vi "foldersfiles.vi"(4 "error in":errorcluster, 7 "path":path) -> (0 "error out":errorcluster, 1 "Array 2":path[](array[path]), 2 "Array":T1(array[cluster]), 3 "path out":path)   [LabVIEW 2010]
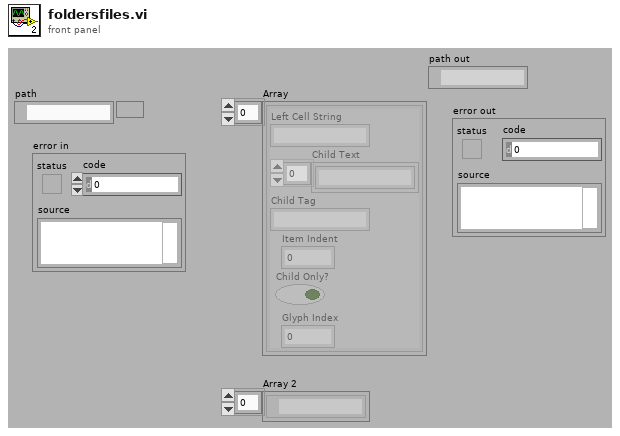
[diagram p1: front panel]
types:
  T1 = cluster{"Left Cell String":string, "Child Text":string[], "Child Tag":string, "Item Indent":i32, "Child Only?":bool, "Glyph Index":i32}[]
  T2 = cluster{"Left Cell String":string, "Child Text":string[], "Child Tag":string, "Item Indent":i32, "Child Only?":bool, "Glyph Index":i32}
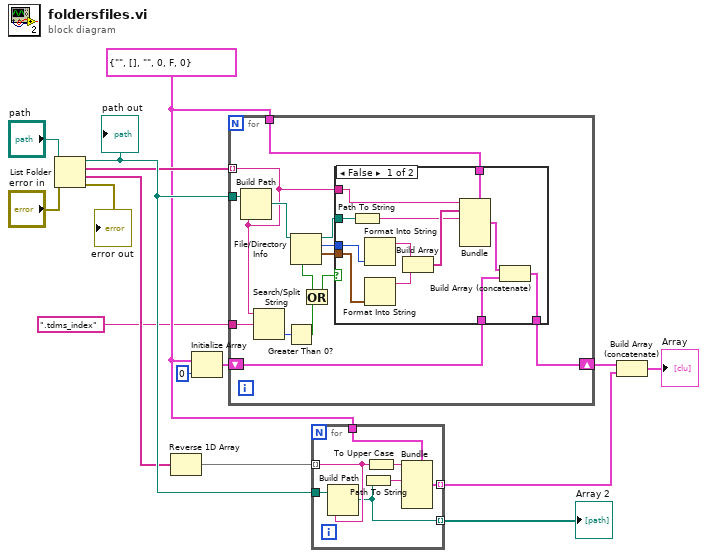
[diagram p0: block diagram]
diagram:
  w4 = T2 {"Left Cell String"="", "Child Text"=[], "Child Tag"="", "Item Indent"=0, "Child Only?"=FALSE, "Glyph Index"=0} ("Item")
  n1 = List Folder(path="path", error in="error in") -> (path out=w14:path, filenames=w6:string[], folder names=w10:string[], error out=→"error out":errorcluster)  [unwired: 2 in]
  "path out" <- w14
  n2 = Reverse 1D Array(array=w10) -> (reversed array=w7:string[])
  n3 = Initialize Array(w4, 0 ("dimension size")) -> (w5:T1)
  n4 = for {
    tunnel: w4 -> [w26]
    tunnel: w6 -> [w23] mode=indexing
    tunnel: w14 -> [w29]
    shift-right: [w16] -> w1
    shift-left: w5 -> [w17]
    tunnel: ".tdms_index" -> [w22]
    n5 = Build Path(base path=w29, name or relative path=w23) -> (appended path=w24:path)
    n6 = Search/Split String(string=w23, search string/char (-)=w22) -> (offset of match=w21:i32)  [unwired: 1 in, 2 out]
    n7 = Greater Than 0?(x=w21) -> (x > 0?=w20:bool)
    n8 = File/Directory Info(path=w24) -> (path out=w25:path, size=w27:i64, last mod=w28:timestamp, shortcut=w19:bool)  [unwired: 1 in, 3 out]
    n9 = Or(x=w19, y=w20) -> (x .or. y?=w18:bool)
    n10 = case shown="False" w18 {
      tunnel: w28 -> [w40 _]
      tunnel: w27 -> [w41 _]
      tunnel: w26 -> [w37 _]
      tunnel: w23 -> [w35 _]
      tunnel: w25 -> [w34 _]
      tunnel: w17 -> [w31 w42]
      tunnel: [w30 w42] -> w16
      frame False {
        n11 = Path To String(path=w34) -> (string=w33:string)
        n12 = Format Into String(w41) -> (resulting string=w38:string)  [unwired: 3 in, 1 out]
        n13 = Format Into String(w40) -> (resulting string=w39:string)  [unwired: 3 in, 1 out]
        n14 = Build Array(w38, w39) -> (w36:string[])
        n15 = Bundle(cluster=w37, "Left Cell String"=w35, "Child Text"=w36, "Child Tag"=w33) -> (w32:T2)  [unwired: 3 in]
        n16 = Build Array (concatenate)(w32, w31) -> (w30:T1)
      }
      frame True {
      }
    }
  }
  n17 = for {
    tunnel: w4 -> [w49]
    tunnel: w7 -> [w47] mode=indexing
    tunnel: w14 -> [w48]
    tunnel: [w46] -> w8 mode=indexing
    tunnel: [w44] -> w11 mode=indexing
    n18 = Build Path(base path=w48, name or relative path=w47) -> (appended path=w44:path)
    n19 = Path To String(path=w44) -> (string=w45:string)
    n20 = To Upper Case(1:w47) -> (0:w43:string)
    n21 = Bundle(cluster=w49, "Left Cell String"=w43, "Child Tag"=w45) -> (w46:T2)  [unwired: 4 in]
  }
  "Array 2" <- w11
  n22 = Build Array (concatenate)(w1, w8) -> (→"Array":T1)
